vi "Reserve ID.vi"(8 "error in (no error)":errorcluster, 10 "Packet Identifier":u16, 11 "Client in":refnum<class "Client.lvclass">) -> (0 "error out":errorcluster, 3 "Client out":refnum<class "Client.lvclass">)   [LabVIEW 2013, in "MQTT Client.lvlib" / "Client.lvclass"]
uses:
  Client.lvclass
  Client.lvclass/Client.ctl
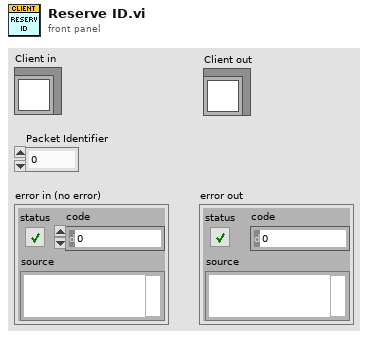
[diagram p1: front panel]
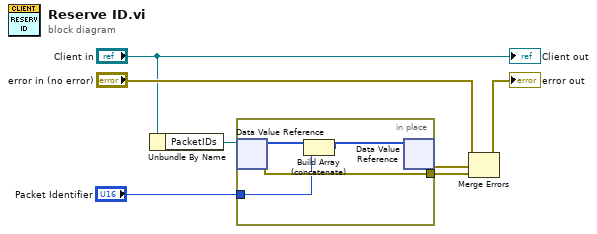
[diagram p0: block diagram]
diagram:
  n1 = Unbundle By Name("Client in") -> ("PacketIDs"=w2:refnum<data-value>)
  n2 = in-place {
    in-place-border: "Packet Identifier" -> [w9]
    in-place-border: [w11] -> w4
    n3 = in-place-dvr #1(w2) -> (w10:u16[], w11:errorcluster)
    n4 = Build Array (concatenate)(w10, w9) -> (w8:u16[])
    n5 = in-place-dvr #1(w8) -> (w5:errorcluster)  [unwired: 1 out]
  }
  n6 = Merge Errors("error in (no error)", w5, w4) -> (→"error out":errorcluster)
  "Client out" <- "Client in"
